vi "ODE Cash Karp 5th Order.vi"(4 "F(X,t) (right sides of the ODE\nas functions of X and t)":string[](array[string]), 5 "X (name of variables)":string[](array[string]), 6 "time":string="t", 7 "time start":dbl format="%.2f", 8 "accuracy":dbl=0.01 min=0.0 format="%.4f", 9 "X0":dbl[](array[numeric]) format="%.2f", 10 "h (step rate)":dbl=0.1 min=0.0 format="%.4f", 11 "time end":dbl=1.0 format="%.2f") -> (0 "error":i32, 1 "ticks":u32, 2 "X Values (solution)":dbl[][](array[numeric]) format="%.2f", 3 "Times":dbl[](array[numeric]) format="%.2f")   [LabVIEW 2020, in "NI_Gmath.lvlib"]
doc: "Solves ordinary differential equations with initial conditions using the Cash Karp method."
uses:
  <vilib>/gmath/NI_Gmath.lvlib
panel:
  out "error message":string
  out "error text":string[](array[string])
  out "error code":i32[](array[numeric])
  # "dX(t)/dt=F(X,t)\nX(0)=X0"
  # "Example:\n\n time start: 0.0 \n time end: 1.0\n h: 0.1\n X0: 1.0 and 1.0 \n time: t\n X: x and y\n F(X,t): sin(t*x)+y and x-y \n accuracy: 0.01"
  # "further error information"
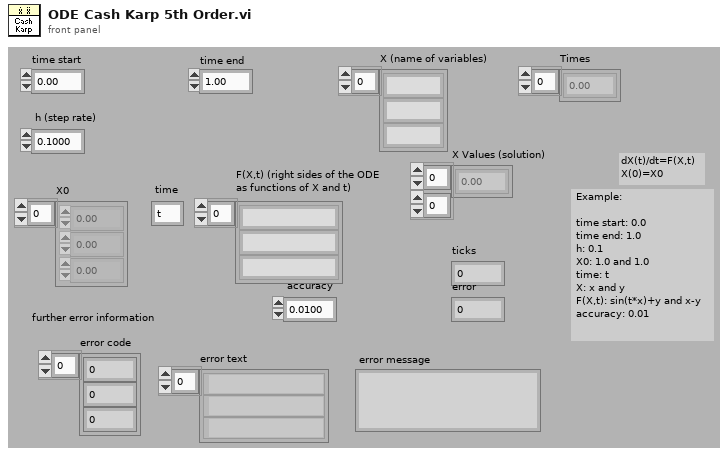
[diagram p1: front panel]
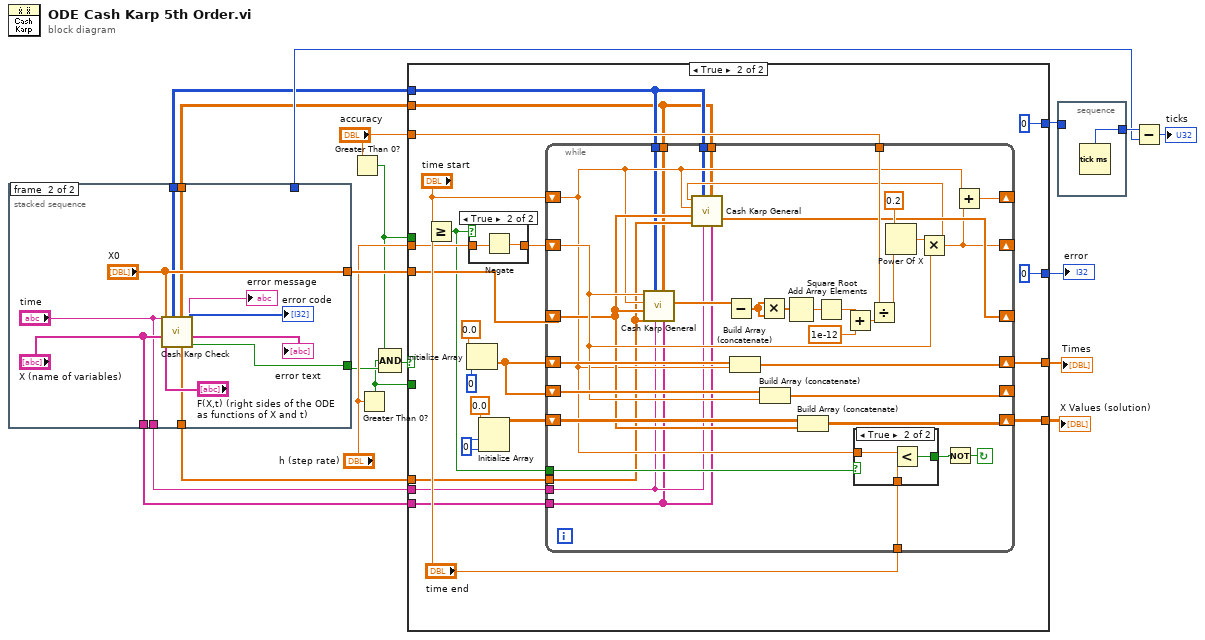
[diagram p0: block diagram]
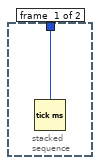
[diagram p2: hidden frame]
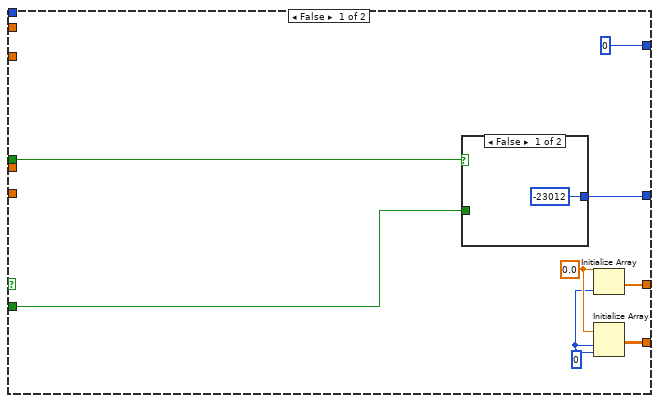
[diagram p3: hidden frame]
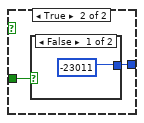
[diagram p4: hidden frame]
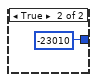
[diagram p5: hidden frame]
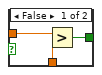
[diagram p6: hidden frame]
diagram:
  n1 = stacked-sequence {
    tunnel: [_ w31] -> w9
    tunnel: [_ "X0"] -> w19
    tunnel: [w20 _] -> w16
    tunnel: [_ w25] -> w5
    tunnel: [_ w24] -> w4
    tunnel: [_ w23] -> w3
    tunnel: [_ "X (name of variables)"] -> w2
    tunnel: [_ "time"] -> w1
    frame #0 {
      n2 = Tick Count (ms)() -> (millisecond timer value=w20:u32)
    }
    frame #1 {
      n3 = call <vilib>:"Cash Karp Check.vi"("F(X,t)"="F(X,t) (right sides of the ODE\nas functions of X and t)", "X"="X (name of variables)", "time"="time", "X(0)"="X0") -> ("system OK"=w31:bool, "error text"=→"error text":string[], "error"=→"error code":i32[], "error message"=→"error message":string, "zero array"=w23:dbl[], "result"=w25:dbl[][], "table"=w24:i32[][][])  [unwired: 1 in]
    }
  }
  n4 = Greater Than 0?(x="accuracy") -> (x > 0?=w7:bool)
  n5 = Greater Than 0?(x="h (step rate)") -> (x > 0?=w6:bool)
  n6 = Compound Arithmetic op=AND(w7, w6, w9) -> (w10:bool)
  n7 = case shown="True" w10 {
    tunnel: w19 -> [_ w64]
    tunnel: [w36 w59] -> w14
    tunnel: [w37 w58] -> w13
    tunnel: [0 0] -> w15
    tunnel: "h (step rate)" -> [_ w52]
    tunnel: "accuracy" -> [_ w55]
    tunnel: [w32 0] -> w8
    tunnel: w7 -> [w34 _]
    tunnel: w6 -> [w33 _]
    tunnel: w5 -> [_ w45]
    tunnel: w4 -> [_ w46]
    tunnel: w3 -> [_ w49]
    tunnel: w2 -> [_ w47]
    tunnel: w1 -> [_ w48]
    frame False {
      w38 = 0
      w39 = 0.0
      n8 = case shown="False" w34 {
        tunnel: w33 -> [_ w42]
        tunnel: [-23012 w41] -> w32
        frame False {
        }
        frame True {
          n9 = case shown="False" w42 {
            tunnel: [-23011 -23010] -> w41
            frame False {
            }
            frame True {
            }
          }
        }
      }
      n10 = Initialize Array(w39, w38) -> (w36:dbl[])
      n11 = Initialize Array(w39, w38, w38) -> (w37:dbl[][])
    }
    frame True {
      w57 = 0
      n12 = Greater Or Equal?(x="time start", y="time end") -> (x >= y?=w50:bool)
      n13 = Initialize Array(0.0, 0) -> (w60:dbl[])
      n14 = case shown="True" w50 {
        tunnel: w52 -> [w108 w110]
        tunnel: [w108 w109] -> w51
        frame False {
        }
        frame True {
          n15 = Negate(x=w110) -> (-x=w109:dbl)
        }
      }
      n16 = Initialize Array(0.0, w57, w57) -> (w63:dbl[][])
      n17 = while {
        tunnel: w50 -> [w78]
        shift-left: w63 -> [w92]
        shift-right: [w89] -> w58
        shift-left: w60 -> [w93]
        shift-right: [w90] -> _
        shift-left: w60 -> [w94]
        shift-right: [w91] -> w59
        tunnel: w55 -> [w97]
        shift-left: w51 -> [w88]
        shift-right: [w76] -> _
        tunnel: "time end" -> [w99]
        shift-left: w64 -> [w83]
        shift-right: [w84] -> _
        shift-left: "time start" -> [w77]
        shift-right: [w75] -> _
        tunnel: w49 -> [w73]
        tunnel: w48 -> [w72]
        tunnel: w47 -> [w71]
        tunnel: w46 -> [w70]
        tunnel: w45 -> [w69]
        tunnel: w46 -> [w68]
        tunnel: w45 -> [w67]
        stop <- w87 continue-if-true
        n18 = call <vilib>:"Cash Karp General.vi"("X"=w71, "result"=w69, "time"=w72, "table"=w70, "zero"=w73, "yn"=w83, "xn"=w77, "h"=w88) -> ("yn2"=w101:dbl[], "yn1"=w100:dbl[])  [unwired: 2 in]
        n19 = Subtract(x=w100, y=w101) -> (x-y=w82:dbl[])
        n20 = Build Array (concatenate)(w94, w77) -> (w91:dbl[])
        n21 = Multiply(x=w82, y=w82) -> (x*y=w81:dbl[])
        n22 = Build Array (concatenate)(w93, w88) -> (w90:dbl[])
        n23 = Add Array Elements(numeric array=w81) -> (sum=w79:dbl)
        n24 = Build Array (concatenate)(w92, w83) -> (w89:dbl[][])
        n25 = Square Root(x=w79) -> (sqrt(x)=w80:dbl)
        n26 = Add(x=w80, y=1e-12) -> (x+y=w85:dbl)
        n27 = case shown="True" w78 {
          tunnel: w77 -> [w104 w107]
          tunnel: [w103 w106] -> w98
          tunnel: w99 -> [w102 w105]
          frame False {
            n28 = Greater?(x=w104, y=w102) -> (0:w103:bool)
          }
          frame True {
            n29 = Less?(x=w107, y=w105) -> (x < y?=w106:bool)
          }
        }
        n30 = Divide(x=w97, y=w85) -> (x/y=w96:dbl)
        n31 = Power Of X(1:w96, 2:0.2) -> (0:w74:dbl)
        n32 = Multiply(x=w74, y=w88) -> (x*y=w76:dbl)
        n33 = call <vilib>:"Cash Karp General.vi"("X"=w71, "result"=w67, "time"=w72, "table"=w68, "zero"=w73, "yn"=w83, "xn"=w77, "h"=w76) -> ("yn2"=w84:dbl[])  [unwired: 2 in, 1 out]
        n34 = Not(x=w98) -> (.not. x?=w87:bool)
        n35 = Add(x=w77, y=w76) -> (x+y=w75:dbl)
      }
    }
  }
  "Times" <- w14
  "X Values (solution)" <- w13
  "error" <- w8
  n36 = stacked-sequence {
    tunnel: [w111] -> w18
    tunnel: w15 -> [_]
    frame #0 {
      n37 = Tick Count (ms)() -> (millisecond timer value=w111:u32)
    }
  }
  n38 = Subtract(x=w18, y=w16) -> (x-y=→"ticks":u32)
